vi "Mass trajectory.vi"() -> ()   [LabVIEW 2024]
panel:
  in  "?":bool
  in  "?":bool
  out "XY Graph":cluster{dbl[], dbl[]}[](graph)
  out "Time (s)":dbl
  out "Current height (m)":dbl
  out "Velocity vector (m/s)":dbl[](array[numeric])
  in  "Launch angle":dbl(slide) scale=0.0..89.0
  in  "Velocity (m/s)":dbl
  in  "Height (m)":dbl
  in  "Mass (kg)":dbl
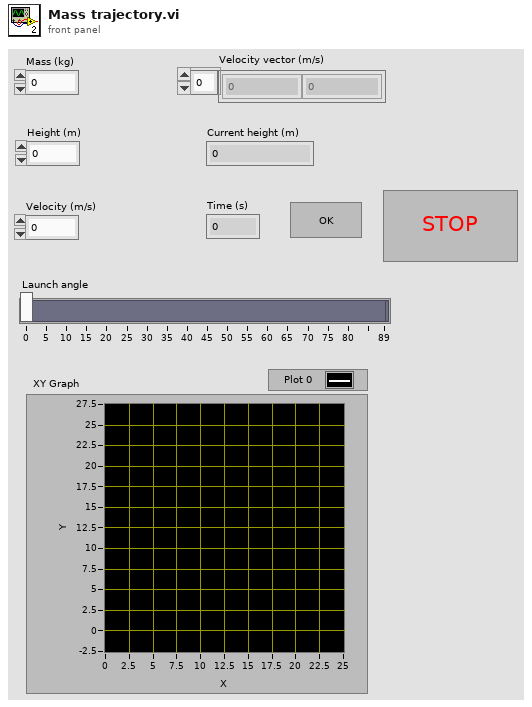
[diagram p1: front panel]
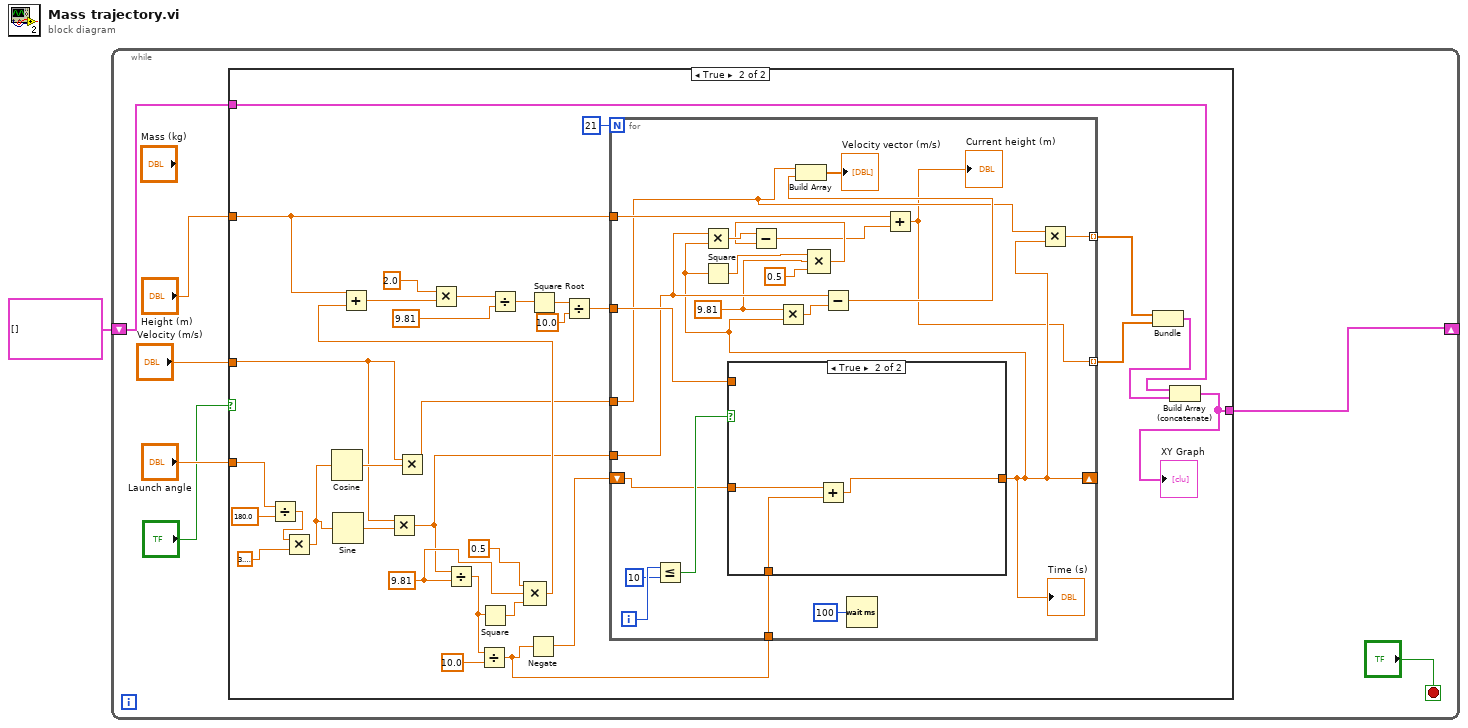
[diagram p0: block diagram]
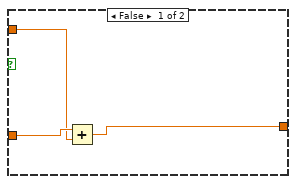
[diagram p3: hidden frame]
diagram:
  n1 = while {
    shift-right: [w2] -> _
    shift-left: cluster{dbl[], dbl[]}[] [] -> [w3]
    stop <- "?" stop-if-true
    n2 = case shown="True" "?" {
      tunnel: "Height (m)" -> [_ w17]
      tunnel: "Velocity (m/s)" -> [_ w16]
      tunnel: "Launch angle" -> [_ w15]
      tunnel: w3 -> [w9 w11]
      tunnel: [w9 w10] -> w2
      frame False {
      }
      frame True {
        w34 = 9.81
        n3 = Divide(x=w15, y=180.0) -> (x/y=w39:dbl)
        n4 = Multiply(x=w39, y=3.141592653589793) -> (x*y=w37:dbl)
        n5 = Cosine(x=w37) -> (cos(x)=w42:dbl)
        n6 = Sine(x=w37) -> (sin(x)=w41:dbl)
        n7 = Multiply(x=w16, y=w41) -> (x*y=w19:dbl)
        n8 = Multiply(x=w16, y=w42) -> (x*y=w18:dbl)
        n9 = Divide(x=w19, y=w34) -> (x/y=w26:dbl)
        n10 = Divide(x=w26, y=10.0) -> (x/y=w23:dbl)
        n11 = Square(x=w26) -> (x^2=w35:dbl)
        n12 = Compound Arithmetic op=MULTIPLY(0.5 ("value"), w34, w35) -> (w33:dbl)
        n13 = Add(x=w17, y=w33) -> (x+y=w32:dbl)
        n14 = Multiply(x=2.0, y=w32) -> (x*y=w29:dbl)
        n15 = Divide(x=w29, y=9.81) -> (x/y=w28:dbl)
        n16 = Negate(x=w23) -> (-x=w24:dbl)
        n17 = Square Root(x=w28) -> (sqrt(x)=w22:dbl)
        n18 = Divide(x=w22, y=10.0) -> (x/y=w20:dbl)
        n19 = for {
          N: 21 -> [_]
          shift-right: [w45] -> _
          shift-left: w24 -> [w60]
          tunnel: w23 -> [w59]
          tunnel: w20 -> [w58]
          tunnel: w19 -> [w54]
          tunnel: w18 -> [w46]
          tunnel: w17 -> [w47]
          tunnel: [w44] -> w14 mode=indexing
          tunnel: [w43] -> w13 mode=indexing
          i -> [w63]
          w51 = 9.81
          n20 = Less Or Equal?(x=w63, y=10) -> (x <= y?=w61:bool)
          n21 = case shown="True" w61 {
            tunnel: w60 -> [w67 w70]
            tunnel: w59 -> [_ w69]
            tunnel: [w65 w68] -> w45
            tunnel: w58 -> [w66 _]
            frame False {
              n22 = Add(x=w67, y=w66) -> (x+y=w65:dbl)
            }
            frame True {
              n23 = Add(x=w70, y=w69) -> (x+y=w68:dbl)
            }
          }
          "Time (s)" <- w45
          n24 = Multiply(x=w54, y=w45) -> (x*y=w53:dbl)
          n25 = Square(x=w45) -> (x^2=w50:dbl)
          n26 = Multiply(x=w51, y=w45) -> (x*y=w57:dbl)
          n27 = Compound Arithmetic op=MULTIPLY(w50, w51, 0.5 ("value")) -> (w49:dbl)
          n28 = Subtract(x=w53, y=w49) -> (x-y=w48:dbl)
          n29 = Subtract(x=w54, y=w57) -> (x-y=w56:dbl)
          n30 = Build Array(w46, w56) -> (→"Velocity vector (m/s)":dbl[])
          n31 = Wait (ms)(milliseconds to wait=u32 100) -> ()  [unwired: 1 out]
          n32 = Add(x=w47, y=w48) -> (x+y=w43:dbl)
          "Current height (m)" <- w43
          n33 = Multiply(x=w46, y=w45) -> (x*y=w44:dbl)
        }
        n34 = Bundle(w14, w13) -> (w12:cluster{dbl[], dbl[]})  [unwired: 1 in]
        n35 = Build Array (concatenate)(w11, w12) -> (w10:cluster{dbl[], dbl[]}[])
        "XY Graph" <- w10
      }
    }
  }
